vi "Vector_place.vi"(11 "vector":cluster{"length":dbl, "angle":dbl, "sense":bool}) -> (3 "x,y":cluster{dbl, dbl})   [LabVIEW 2024]
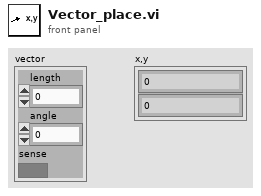
[diagram p1: front panel]
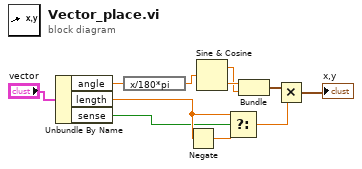
[diagram p0: block diagram]
diagram:
  n1 = Unbundle By Name("vector") -> ("angle"=w11:dbl, "length"=w3:dbl, "sense"=w1:bool)
  n2 = expression code="x/180*pi"(w11) -> (w7:dbl)
  n3 = Negate(x=w3) -> (-x=w4:dbl)
  n4 = Sine & Cosine(0:w7) -> (1:w8:dbl, 2:w9:dbl)
  n5 = Select(t=w3, s=w1, f=w4) -> (s? t:f=w2:dbl)
  n6 = Bundle(w9, w8) -> (w10:cluster{dbl, dbl})  [unwired: 1 in]
  n7 = Multiply(x=w10, y=w2) -> (x*y=→"x,y":cluster{dbl, dbl})
